vi "QI_OpenCam.vi"(8 "error in (no error)":errorcluster, 10 "Camera ID":u32, 11 "path to dll":path) -> (0 "error out":errorcluster, 1 "Open Cam Error":i32, 3 "Camera Handle":u32)   [LabVIEW 2014]
panel:
  in  "handle":u32
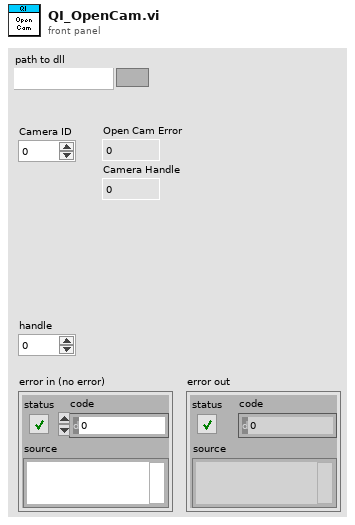
[diagram p1: front panel]
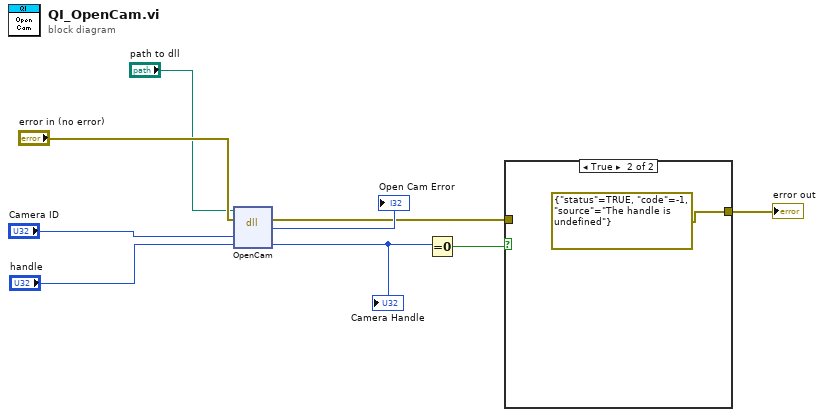
[diagram p0: block diagram]
diagram:
  n1 = dll-call lib="C:/Users/appli/Documents/Aline/octo-labview/QImaging/Release/QImaging.dll" fn="OpenCam"(path in="path to dll", error in="error in (no error)", "cameraid"="Camera ID", "handle"="handle") -> (error out=w3:errorcluster, "return type"=→"Open Cam Error":i32, "handle"=w5:u32)  [unwired: 2 in, 1 out]
  "Camera Handle" <- w5
  n2 = Equal To 0?(x=w5) -> (x = 0?=w4:bool)
  n3 = case shown="True" w4 {
    tunnel: w3 -> [w10 _]
    tunnel: [w10 errorcluster {"status"=TRUE, "code"=-1, "source"="The handle is undefined"} ("error out")] -> w2
    frame False {
    }
    frame True {
    }
  }
  "error out" <- w2
